vi "Flatten Names.vi"   [LabVIEW 2020, in "SLSC.lvlib"]
doc: "Converts an array of names into a comma-delimited list of names."
uses:
  <vilib>/SLSC/SLSC.lvlib
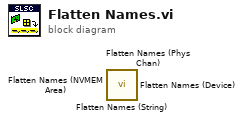
[diagram p0: block diagram]
diagram:
  n1 = call <vilib>:"Flatten Names (String).vi"() -> ()  [unwired: 14 in, 2 out]
  n2 = call <vilib>:"Flatten Names (Phys Chan).vi"() -> ()  [unwired: 14 in, 2 out]
  n3 = call <vilib>:"Flatten Names (NVMEM Area).vi"() -> ()  [unwired: 14 in, 2 out]
  n4 = call <vilib>:"Flatten Names (Device).vi"() -> ()  [unwired: 14 in, 2 out]
